vi "Apply Data To Tree.vi"(6 "Child Position":i32=-1, 8 "error in (no error)":errorcluster, 9 "Tree Item In":T1, 10 "Tree In":refnum<class "Tree.lvclass">, 11 "Tree Data Folder in":refnum<class "Tree Data Folder.lvclass">) -> (0 "error out":errorcluster, 2 "Tree Out":refnum<class "Tree.lvclass">, 3 "Tree Data Folder out":refnum<class "Tree Data Folder.lvclass">)   [LabVIEW 2024, in "Tree Data Folder.lvclass"]
uses:
  Tree Data Folder.lvclass
  Tree/Type Def/Tree Item.ctl
  Tree/Tree.lvclass
  Tree/Tree.lvclass/Tree.ctl
  Tree Data Folder.lvclass/Tree Data Folder.ctl
  Tree/Public Data/Read Root Tag.vi
  Composite Tree Data/Composite Tree Data.lvclass
  Tree Data File/Tree Data File.lvclass
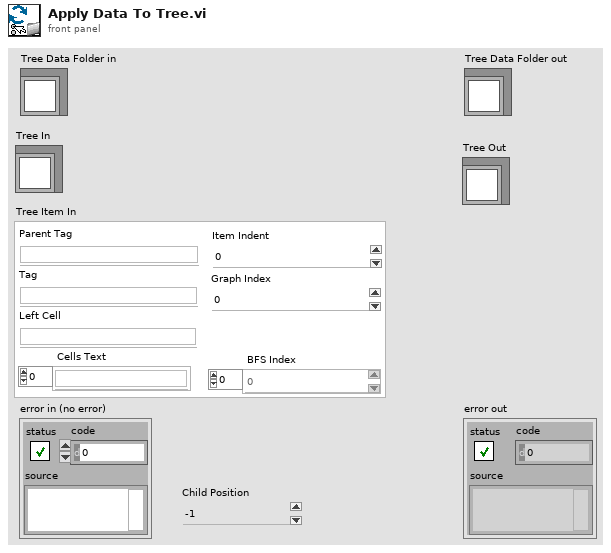
[diagram p1: front panel]
types:
  T1 = typedef "Tree Item.ctl" = cluster{"Parent Tag":string, "Tag":string, "Left Cell":string, "Cells Text":string[], "BFS Index":i32[], "Graph Index":i32, "Item Indent":i32}
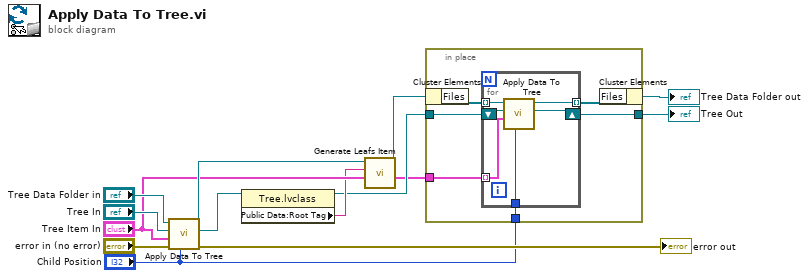
[diagram p0: block diagram]
diagram:
  n1 = call-parent "Apply Data To Tree.vi"("Child Position"="Child Position", "error in (no error)"="error in (no error)", "Tree Item In"="Tree Item In", "Tree In"="Tree In", "Composite Tree Data in"="Tree Data Folder in") -> ("error out"=→"error out":errorcluster, "Tree Out"=w6:refnum<class "Tree.lvclass">, "Composite Tree Data out"=w9:refnum<class "Tree Data Folder.lvclass">)  [unwired: 4 in]
  n2 = property class="Tree.lvclass"(reference=w6) -> (reference out=w3:refnum<class "Tree.lvclass">, "Public Data:Root Tag"=w5:string)  [unwired: 1 in, 1 out]
  n3 = call-dynamic "Generate Leafs Item.vi"("Tree Item In"="Tree Item In", "Root Tag In"=w5, "Tree Data Folder In"=w9) -> ("Leafs Item Out"=w2:T1[], "Tree Data Folder Out"=w4:refnum<class "Tree Data Folder.lvclass">)  [unwired: 6 in, 1 out]
  n4 = in-place {
    in-place-border: w3 -> [w18]
    in-place-border: [w17] -> w10
    in-place-border: w2 -> [w16]
    in-place-border: "Child Position" -> [w15]
    n5 = in-place-cluster #1(w4) -> ("Files"=w20:refnum<class "Tree Data File.lvclass">[])
    n6 = for {
      tunnel: w20 -> [w26] mode=indexing
      tunnel: [w25] -> w19 mode=indexing
      shift-right: [w23] -> w17
      shift-left: w18 -> [w24]
      tunnel: w16 -> [w22] mode=indexing
      tunnel: w15 -> [w21]
      n7 = call-dynamic "Apply Data To Tree.vi"("Child Position"=w21, "Tree Item In"=w22, "Tree In"=w24, "Composite Tree Data in"=w26) -> ("Tree Out"=w23:refnum<class "Tree.lvclass">, "Composite Tree Data out"=w25:refnum<class "Tree Data File.lvclass">)  [unwired: 5 in, 1 out]
    }
    n8 = in-place-cluster #1("Files"=w19) -> (→"Tree Data Folder out":refnum<class "Tree Data Folder.lvclass">)
  }
  "Tree Out" <- w10
